vi "FTW-ActorTemplate.vi"(0 "Actor Instance Configuration":string="{\n  \"Identity\": \"ActorName\",\n  \"InboxAddress\": \"tcp://127.0.0.1:*\",\n  \"SupervisorAddress\": \"\",\n  \"DebugEnableInboxLogging\": false,\n  \"DebugEnableJobLogging\": false,\n  \"DebugShowPanel\": false\n}", 11 "ErrorIn":errorcluster) -> (15 "Error":errorcluster)   [LabVIEW 2014]
uses:
  src/actor/instance/FTW-Actor-Instance.lvclass
panel:
  # "Inputs"
  # "Outputs"
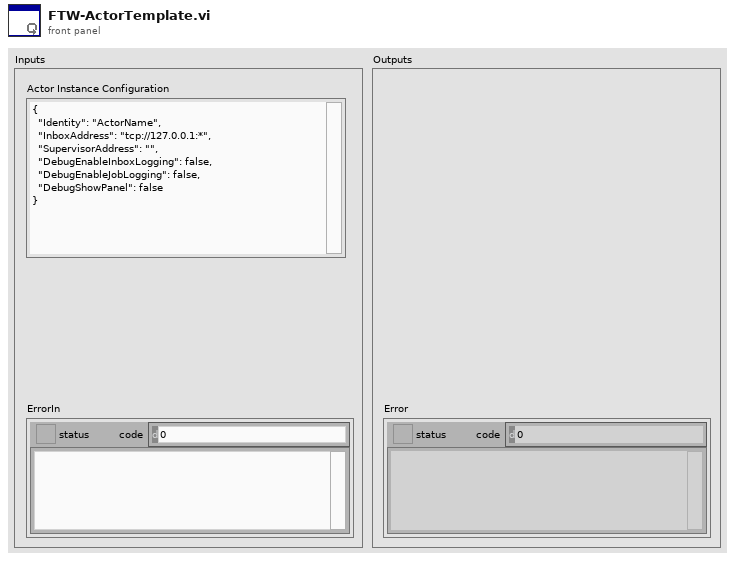
[diagram p1: front panel]
types:
  T1 = cluster{"Incoming Request":refnum<event-registration>}
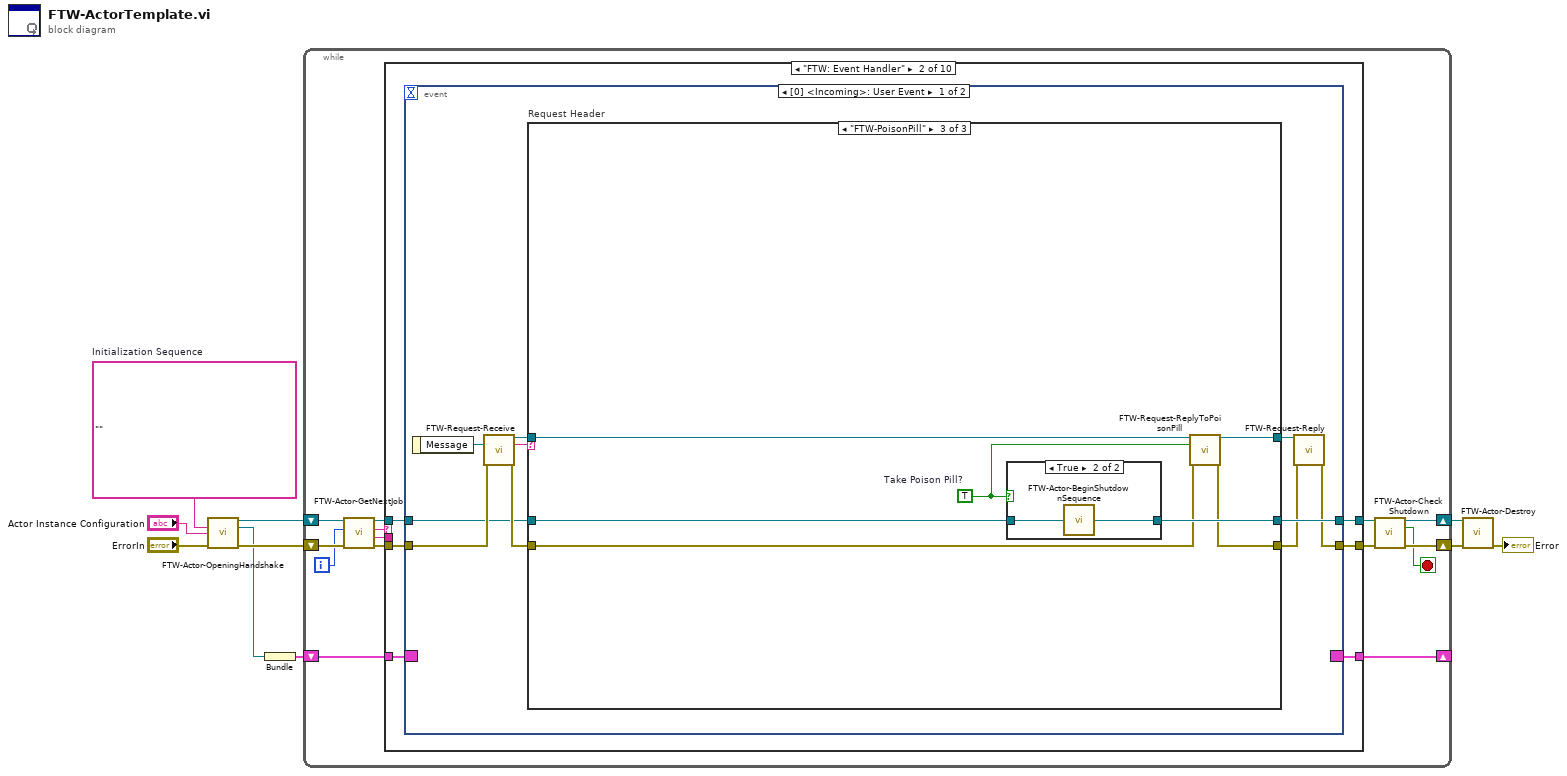
[diagram p0: block diagram]
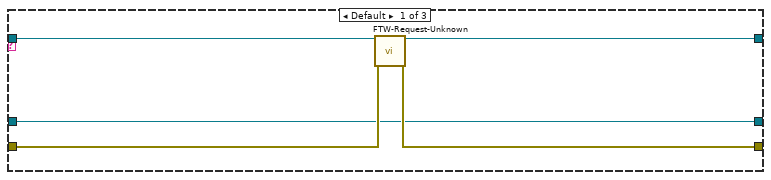
[diagram p3: hidden frame]
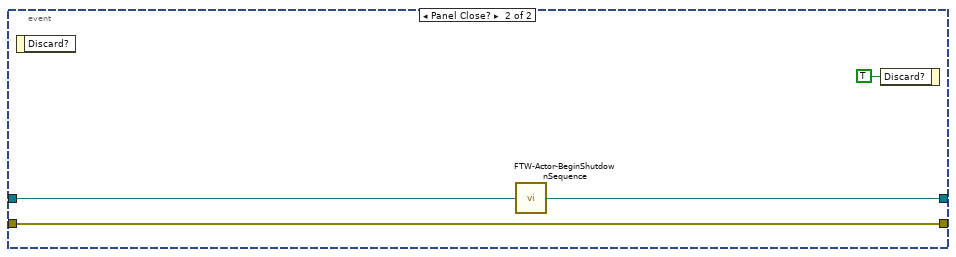
[diagram p6: hidden frame]
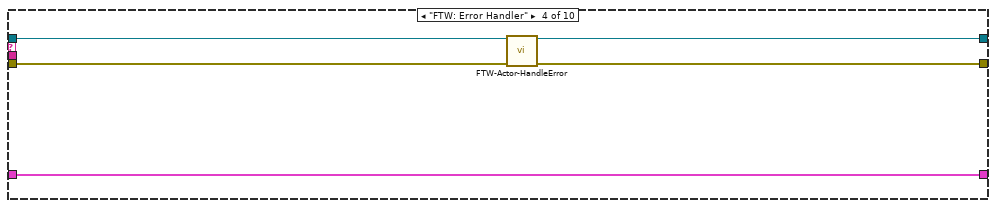
[diagram p8: hidden frame]
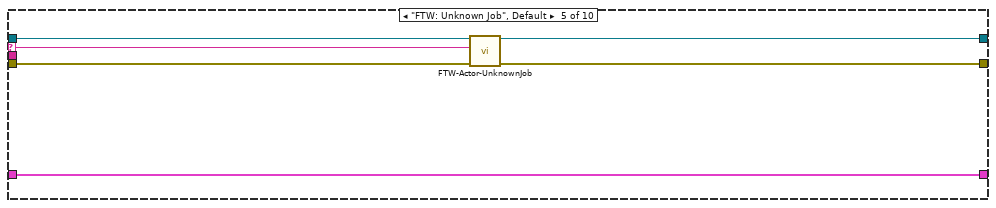
[diagram p9: hidden frame]
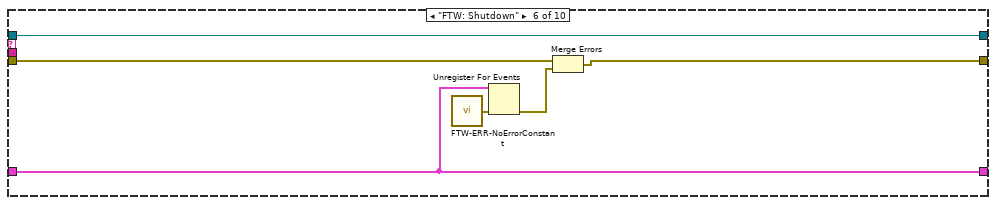
[diagram p10: hidden frame]
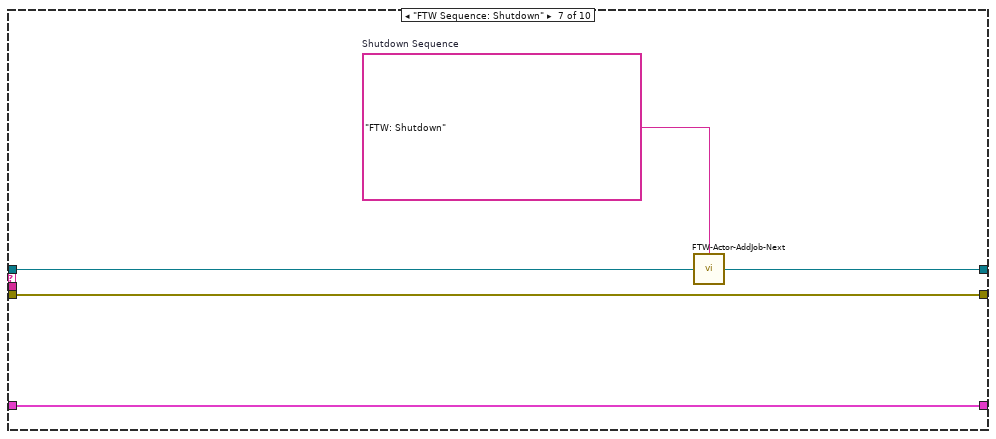
[diagram p11: hidden frame]
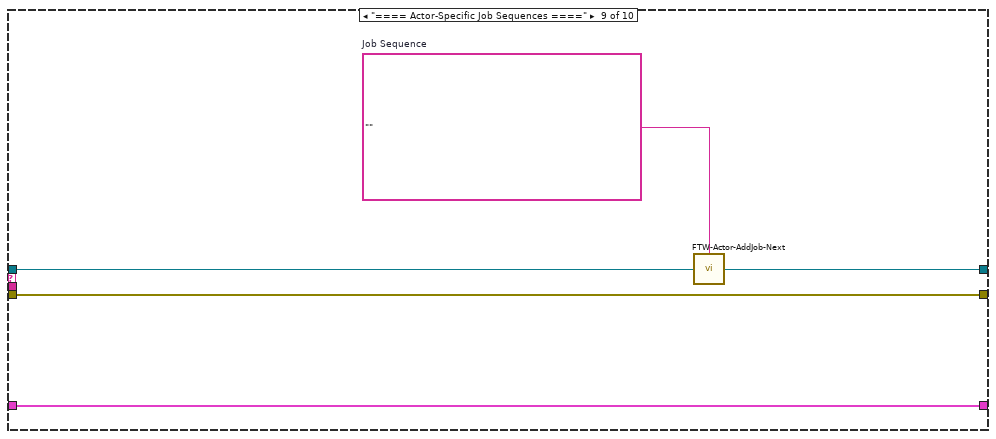
[diagram p13: hidden frame]
diagram:
  w5 = ""  # Initialization Sequence
  n1 = call "FTW-Actor-OpeningHandshake.vi"("Initialization Job Sequence"=w5, "Actor Instance Configuration"="Actor Instance Configuration", "error in"="ErrorIn") -> ("FTW Actor Instance"=w10:refnum<class "FTW-Actor-Instance.lvclass">, "Incoming Request"=w1:refnum<event-registration>, "error out"=w6:errorcluster)  [unwired: 10 in]
  n2 = Bundle("Incoming Request"=w1) -> (w3:T1)  [unwired: 1 in]
  n3 = while {
    shift-right: [w14] -> w8
    shift-left: w6 -> [w21]
    shift-right: [w11] -> _
    shift-left: w3 -> [w24]
    shift-right: [w16] -> w9
    shift-left: w10 -> [w23]
    i -> [w12]
    stop <- w13 stop-if-true
    n4 = call "FTW-Actor-GetNextJob.vi"("error in"=w21, "Jobs Performed"=w12, "FTW Actor Instance"=w23) -> ("error out"=w20:errorcluster, "Job Data"=w18:string, "Job Name"=w19:string, "FTW Actor Instance out"=w22:refnum<class "FTW-Actor-Instance.lvclass">)  [unwired: 5 in]
    n5 = case shown="\"FTW: Event Handler\"" w19 {
      selector: w19 -> [_ _ _ _ w74 _ _ _ _ _]
      tunnel: [w26 w33 w66 w69 w77 w84 w89 w92 w97 w101] -> w15
      tunnel: w20 -> [w26 w32 w66 w71 w78 w85 w89 w92 w97 w101]
      tunnel: w24 -> [w27 w28 w68 w73 w79 w81 w90 w93 w98 w100]
      tunnel: [w27 w31 w68 w73 w79 w81 w90 w93 w98 w100] -> w11
      tunnel: w18 -> [_ _ _ _ _ _ _ _ _ _]
      tunnel: [w25 w30 w67 w70 w75 w82 w87 w91 w95 w99] -> w17
      tunnel: w22 -> [w25 w29 w67 w72 w76 w82 w88 w91 w96 w99]
      frame "==== Featherweight Framework Jobs ====" {
      }
      frame "FTW: Event Handler" {
        n6 = event shown="[0] <Incoming>: User Event" {
          selector: w28 -> [_ _]
          dyn-events: [_ _] -> w31
          timeout: _ -> [_ _]
          tunnel: [w37 w64] -> w33
          tunnel: w32 -> [w42 w64]
          tunnel: [w41 w62] -> w30
          tunnel: w29 -> [w40 w63]
          event User Event {
            n7 = event-data() -> ("Message"=w34:refnum<queue>)  [unwired: 1 in]
            n8 = call "FTW-Request-Receive.vi"("MessagePipe"=w34, "error in"=w42) -> ("Request"=w38:refnum<data-value>, "Request Header"=w39:string, "error out"=w43:errorcluster)  [unwired: 11 in]
            n9 = case "Request Header" shown="\"FTW-PoisonPill\"" w39 {
              tunnel: [w47 w49 w53] -> w36
              tunnel: w43 -> [w48 w49 w54]
              tunnel: [w45 w51 w58] -> w41
              tunnel: w40 -> [w45 w51 w57]
              tunnel: w38 -> [w46 w50 w56]
              tunnel: [w44 w50 w55] -> w35
              frame Default {
                n10 = call "FTW-Request-Unknown.vi"("Request"=w46, "error in"=w48) -> ("Request out"=w44:refnum<data-value>, "error out"=w47:errorcluster)  [unwired: 12 in]
              }
              frame "FTW-ActorStatus" {
              }
              frame "FTW-PoisonPill" {
                w52 = TRUE  # Take Poison Pill?
                n11 = case shown="True" w52 {
                  tunnel: [w59 w61] -> w58
                  tunnel: w57 -> [w59 w60]
                  frame False {
                  }
                  frame True {
                    n12 = call "FTW-Actor-BeginShutdownSequence.vi"("FTW Actor Instance"=w60) -> ("FTW Actor Instance out"=w61:refnum<class "FTW-Actor-Instance.lvclass">)  [unwired: 3 in]
                  }
                }
                n13 = call "FTW-Request-ReplyToPoisonPill.vi"("Poison Pill Request"=w56, "Shutting Down?"=w52, "error in"=w54) -> ("Poison Pill Response"=w55:refnum<data-value>, "error out"=w53:errorcluster)  [unwired: 11 in]
              }
            }
            n14 = call "FTW-Request-Reply.vi"("Request"=w35, "error in"=w36) -> ("error out"=w37:errorcluster)  [unwired: 13 in]
          }
          event Panel Close? {
            n15 = event-data() -> ()  [unwired: 1 in, 1 out]
            n16 = call "FTW-Actor-BeginShutdownSequence.vi"("FTW Actor Instance"=w63) -> ("FTW Actor Instance out"=w62:refnum<class "FTW-Actor-Instance.lvclass">)  [unwired: 3 in]
            n17 = event-data("Discard?"=TRUE) -> ()  [unwired: 1 in, 1 out]
          }
        }
      }
      frame "FTW: Failure to Launch" {
      }
      frame "FTW: Error Handler" {
        n18 = call-dynamic "FTW-Actor-HandleError.vi"("FTW Actor Instance"=w72, "error in"=w71) -> ("FTW Actor Instance out"=w70:refnum<class "FTW-Actor-Instance.lvclass">, "error out"=w69:errorcluster)  [unwired: 11 in, 1 out]
      }
      frame "FTW: Unknown Job", Default {
        n19 = call-dynamic "FTW-Actor-UnknownJob.vi"("FTW Actor Instance"=w76, "Unknown Job"=w74, "error in"=w78) -> ("FTW Actor Instance out"=w75:refnum<class "FTW-Actor-Instance.lvclass">, "error out"=w77:errorcluster)  [unwired: 11 in]
      }
      frame "FTW: Shutdown" {
        n20 = call "FTW-ERR-NoErrorConstant.vi"() -> ("no error"=w80:errorcluster)
        n21 = Unregister For Events(event registration refnum=w81, error in=w80) -> (error out=w83:errorcluster)
        n22 = Merge Errors(w85, w83) -> (w84:errorcluster)
      }
      frame "FTW Sequence: Shutdown" {
        w86 = "FTW: Shutdown"  # Shutdown Sequence
        n23 = call "FTW-Actor-AddJob-Next.vi"("Add Next in Job Queue"=w86, "FTW Actor Instance"=w88) -> ("FTW Actor Instance out"=w87:refnum<class "FTW-Actor-Instance.lvclass">)  [unwired: 2 in]
      }
      frame "==== Actor-Specific Static Dependencies ====" {
      }
      frame "==== Actor-Specific Job Sequences ====" {
        w94 = ""  # Job Sequence
        n24 = call "FTW-Actor-AddJob-Next.vi"("Add Next in Job Queue"=w94, "FTW Actor Instance"=w96) -> ("FTW Actor Instance out"=w95:refnum<class "FTW-Actor-Instance.lvclass">)  [unwired: 2 in]
      }
      frame "==== Actor-Specific Jobs ====" {
      }
    }
    n25 = call "FTW-Actor-CheckShutdown.vi"("FTW Actor Instance"=w17, "error in"=w15) -> ("FTW Actor Instance out"=w16:refnum<class "FTW-Actor-Instance.lvclass">, "Shutdown?"=w13:bool, "error out"=w14:errorcluster)  [unwired: 11 in]
  }
  n26 = call-dynamic "FTW-Actor-Destroy.vi"("FTW Actor Instance"=w9, "error in"=w8) -> ("error out"=→"Error":errorcluster)  [unwired: 13 in]
